vi "SPI_TEST.vi"() -> ()   [LabVIEW 2014]
uses:
  navX-MXP Library/COMMON/TypeDefs/navX YPRH Data.ctl
  navX-MXP Library/COMMON/TypeDefs/navX Quaternion Data.ctl
  navX-MXP Library/COMMON/TypeDefs/navX Vector Data.ctl
  navX-MXP Library/COMMON/TypeDefs/navX Status Data.ctl
  navX-MXP Library/COMMON/TypeDefs/navX NAVX_OP_STATUS.ctl
  navX-MXP Library/COMMON/TypeDefs/navX NAVX_CAL_STATUS.ctl
  navX-MXP Library/COMMON/TypeDefs/navX NAVX_SENSOR_STATUS.ctl
  <vilib>/Platform/TimedLoop/XDataNode/timing_clust.ctl
  <vilib>/Platform/TimedLoop/XDataNode/nitl_modes.ctl
  <vilib>/Platform/TimedLoop/XDataNode/wakeup.ctl
  <vilib>/platform/TimedLoop/XDataNode/XDataNode.xnode
  navX-MXP Library/navX-MXP IMU.lvlib
  <vilib>/Platform/TimedLoop/XDataNode/XDNodeRunTimeDep.lvlib
panel:
  out "Fused Heading":dbl
  out "Status":T1={"Update Rate Hz"=0, "Accelerometer Full-Scale Range"=0, "Gyro Full-Scale Range"=0, "NAVX_OP_STATUS"=0, "NAVX_CAL_STATUS"=0, "NAVX_SELFTEST_STATUS"=80, "NAVX_SENSOR_STATUS"={"MOVING"=FALSE, "YAW_STABLE"=FALSE, "MAG_DISTURBANCE"=FALSE, "ALTITUDE_VALID"=FALSE, "SEALEVEL_PRESS_SET"=FALSE, "FUSED_HEADING_VALID"=FALSE}} {"NAVX_OP_STATUS" items=["INITIALIZING", "SELFTEST_IN_PROGRESS", "ERROR", "IMU_AUTOCAL_IN_PROGRESS", "NORMAL"]; "NAVX_CAL_STATUS" items=["IMU_CAL_STATE_MASK"=3, "IMU_CAL_INPROGRESS"=0, "IMU_CAL_ACCUMULATE"=1, "IMU_CAL_COMPLETE"=2, "MAG_CAL_COMPLETE"=4, "BARO_CAL_COMPLETE"=8]}
  out "RawMag":T5
  out "RawGyro":T5
  out "RawAccel":T5
  in  "Zero":bool
  out "Quaternion":T6
  out "YPRH":T7
  out "Acceleration":T5(graph)
  out "Valid?":bool
  in  "stop":bool
  out "Opened":bool
  in  "Update Rate (4Hz-60Hz)":u8=40
  # "SPI"
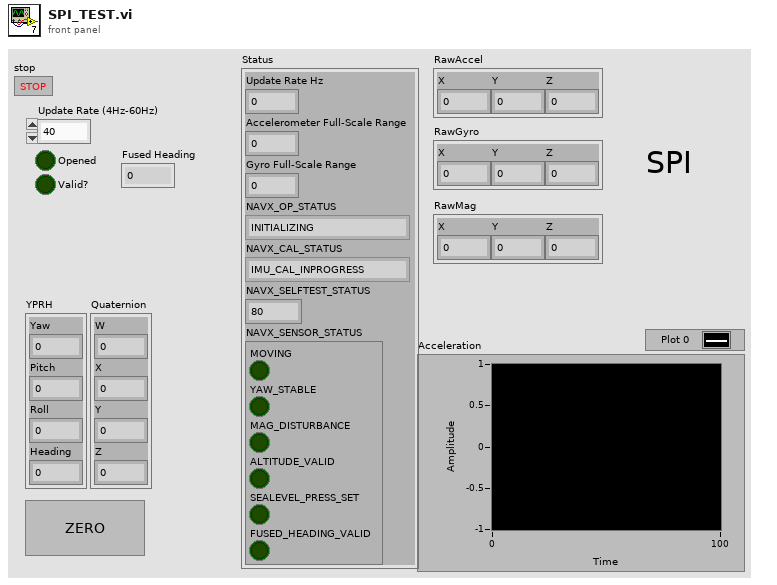
[diagram p1: front panel]
types:
  T1 = typedef "navX-MXP IMU.lvlib/navX Status Data.ctl" = cluster{"Update Rate Hz":u8, "Accelerometer Full-Scale Range":u8, "Gyro Full-Scale Range":u16, "NAVX_OP_STATUS":T2, "NAVX_CAL_STATUS":T3, "NAVX_SELFTEST_STATUS":u8, "NAVX_SENSOR_STATUS":T4}
  T2 = typedef "navX-MXP IMU.lvlib/navX NAVX_OP_STATUS.ctl" = u8
  T3 = typedef "navX-MXP IMU.lvlib/navX NAVX_CAL_STATUS.ctl" = u8
  T4 = typedef "navX-MXP IMU.lvlib/navX NAVX_SENSOR_STATUS.ctl" = cluster{"MOVING":bool, "YAW_STABLE":bool, "MAG_DISTURBANCE":bool, "ALTITUDE_VALID":bool, "SEALEVEL_PRESS_SET":bool, "FUSED_HEADING_VALID":bool}
  T5 = typedef "navX-MXP IMU.lvlib/navX Vector Data.ctl" = cluster{"X":dbl, "Y":dbl, "Z":dbl}
  T6 = typedef "navX-MXP IMU.lvlib/navX Quaternion Data.ctl" = cluster{"W":dbl, "X":dbl, "Y":dbl, "Z":dbl}
  T7 = typedef "navX-MXP IMU.lvlib/navX YPRH Data.ctl" = cluster{"Yaw":dbl, "Pitch":dbl, "Roll":dbl, "Heading":dbl}
  T8 = typedef "navX-MXP IMU.lvlib/navX SPI DevRef.ctl" = cluster{"SPIDevRef":T9, "Board Information":T12, "Status":T1, "Offsets":cluster{"Yaw":dbl, "Quat W":dbl, "Quat X":dbl, "Quat Y":dbl, "Quat Z":dbl}, "Update Rate (4Hz-60Hz)":u8, "refnum name":string, "error":errorcluster}
  T9 = typedef "WPI_SPIDevRef.ctl" = cluster{"DevStatus":errorcluster, "Handle":i32, "Controller":T10, "SPI Bus":T11}
  T10 = typedef "FPGA_TypedefDigitalModule.ctl" = enum16{"Controller 1"}
  T11 = typedef "spi_bus.ctl" = enum16{"SPI On-Board, CS0", "SPI On-Board, CS1", "SPI On-Board, CS2", "SPI On-Board, CS3", "SPI MXP", "Invalid"}
  T12 = typedef "navX-MXP IMU.lvlib/navX Board Information.ctl" = cluster{"WhoAmI (50 | 0x32)":u8, "Board Revision":u8, "Firmware Major Version":u8, "Firmware Minor Version":u8}
  T13 = typedef "XDNodeRunTimeDep.lvlib/timing_clust.ctl" = cluster{"Expected End [f-1]":u64, "Actual End [f-1]":u64, "Finished Late? [f-1]":bool, "Expected End [i-1]":u64, "Actual End [i-1]":u64, "Finished Late? [i-1]":bool, "Expected Start [i]":u64, "Actual Start [i]":u64, "Expected Start [f]":u64, "Actual Start [f]":u64, "Source Name":string, "Structure Name":string, "Period":i64, "Deadline":i64, "Offset":i64, "Start":i64, "Priority":i32, "Timeout":i32, "Mode":T14, "Wakeup Reason":T15, "Error":errorcluster, "Source Type":string, "Secondary Source Type":string, "Global End Time":u64, "Global Start Time":u64, "Frame Duration":u64, "Iteration Duration":u64, "Assigned CPU":i32, "I/O Scan Engine Mode":u32}
  T14 = typedef "XDNodeRunTimeDep.lvlib/nitl_modes.ctl" = enum32{"No Change", "Process missed periods, maintain original phase", "Discard missed periods, maintain original phase", "Process missed periods, ignore original phase", "Discard missed periods, ignore original phase"}
  T15 = typedef "XDNodeRunTimeDep.lvlib/wakeup.ctl" = enum32{"Normal", "Aborted", "Asynchronous wakeup", "Timing source error", "Timed loop error", "Timeout"}
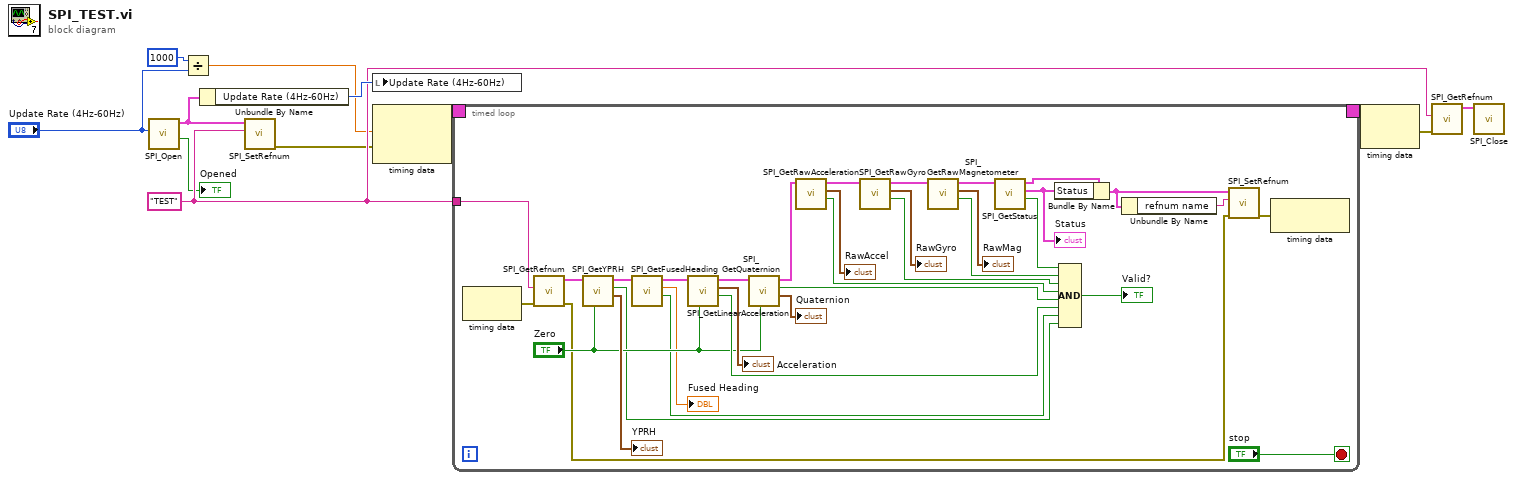
[diagram p0: block diagram]
diagram:
  w7 = "TEST" ("refnum name")
  n1 = call "SPI_Open.vi"("Update Rate (4Hz-60Hz)"="Update Rate (4Hz-60Hz)") -> ("Opened"=→"Opened":bool, "navX DevRef"=w3:T8)  [unwired: 8 in, 1 out]
  n2 = Divide(x=1000, y="Update Rate (4Hz-60Hz)") -> (x/y=w6:dbl)
  n3 = Unbundle By Name(w3) -> ("Update Rate (4Hz-60Hz)"=w8:u8)
  n4 = call "SPI_SetRefnum.vi"("refnum name"=w7, "navX DevRef"=w3) -> ("error out"=w5:errorcluster)  [unwired: 8 in, 1 out]
  n5 = local write "Update Rate (4Hz-60Hz)"(w8) -> ()
  n6 = node-c288(w6, w5) -> (w12:T13)
  n7 = timed-loop {
    timing: w12 -> [_]
    timing-out: [_] -> w11
    tunnel: w7 -> [w32]
    stop <- "stop" stop-if-true
    n8 = node-c288() -> (w30:errorcluster)  [unwired: 1 in]
    n9 = call "SPI_GetRefnum.vi"("error in (no error)"=w30, "refnum name"=w32) -> ("error out"=w31:errorcluster, "navX DevRef"=w33:T8)  [unwired: 8 in]
    n10 = call "SPI_GetYPRH.vi"("Zero"="Zero", "navX DevRef"=w33) -> ("YPRH"=→"YPRH":T7, "Valid?"=w15:bool, "navX DevRef"=w17:T8)  [unwired: 7 in]
    n11 = call "SPI_GetFusedHeading.vi"("navX DevRef"=w17) -> ("Valid?"=w14:bool, "Fused Heading"=→"Fused Heading":dbl, "navX DevRef"=w16:T8)  [unwired: 8 in]
    n12 = call "SPI_GetLinearAcceleration.vi"("Zero"="Zero", "navX DevRef"=w16) -> ("Valid?"=w44:bool, "Acceleration"=→"Acceleration":T5, "navX DevRef"=w42:T8)  [unwired: 7 in]
    n13 = call "SPI_GetQuaternion.vi"("Zero"="Zero", "navX DevRef"=w42) -> ("Quaternion"=→"Quaternion":T6, "Valid?"=w41:bool, "navX DevRef"=w28:T8)  [unwired: 7 in]
    n14 = call "SPI_GetRawAcceleration.vi"("navX DevRef"=w28) -> ("Valid?"=w24:bool, "Vector"=→"RawAccel":T5, "navX DevRef"=w27:T8)  [unwired: 8 in]
    n15 = call "SPI_GetRawGyro.vi"("navX DevRef"=w27) -> ("Valid?"=w23:bool, "Vector"=→"RawGyro":T5, "navX DevRef"=w26:T8)  [unwired: 8 in]
    n16 = call "SPI_GetRawMagnetometer.vi"("navX DevRef 2"=w26) -> ("Valid?"=w22:bool, "Vector"=→"RawMag":T5, "navX DevRef"=w25:T8)  [unwired: 8 in]
    n17 = call "SPI_GetStatus.vi"("navX DevRef"=w25) -> ("Valid?"=w21:bool, "Status"=w36:T1, "navX DevRef"=w37:T8)  [unwired: 8 in]
    "Status" <- w36
    n18 = Bundle By Name(cluster=w37, "Status"=w36) -> (w34:T8)
    n19 = Compound Arithmetic op=AND(w21, w22, w23, w24, w41, w44, w14, w15) -> (→"Valid?":bool)
    n20 = Unbundle By Name(w34) -> ("refnum name"=w35:string)
    n21 = call "SPI_SetRefnum.vi"("error in (no error)"=w31, "refnum name"=w35, "navX DevRef"=w34) -> ("error out"=w29:errorcluster)  [unwired: 7 in, 1 out]
    n22 = node-c288(w29) -> ()  [unwired: 1 out]
  }
  n23 = node-c288(w11) -> (w4:errorcluster)
  n24 = call "SPI_GetRefnum.vi"("error in (no error)"=w4, "refnum name"=w7) -> ("navX DevRef"=w2:T8)  [unwired: 8 in, 1 out]
  n25 = call "SPI_Close.vi"("navX DevRef"=w2) -> ()  [unwired: 10 in, 1 out]
